vi "Add Item to Tree.vi"(6 "Display Text Override":string, 8 "error in (no error)":errorcluster, 9 "Parent Tag":string, 10 "Data Item":refnum<class "Data Item.lvclass">, 11 "Tree Manager in":refnum<class "Tree Manager.lvclass">) -> (0 "error out":errorcluster, 2 "New Tag":string, 3 "Tree Manager out":refnum<class "Tree Manager.lvclass">)   [LabVIEW 2026, in "VILab.lvlib" / "Tree Manager.lvclass"]
uses:
  Tree Manager.lvclass
  Data Item/Data Item.lvclass
  Tree Manager.lvclass/Tree Manager.ctl
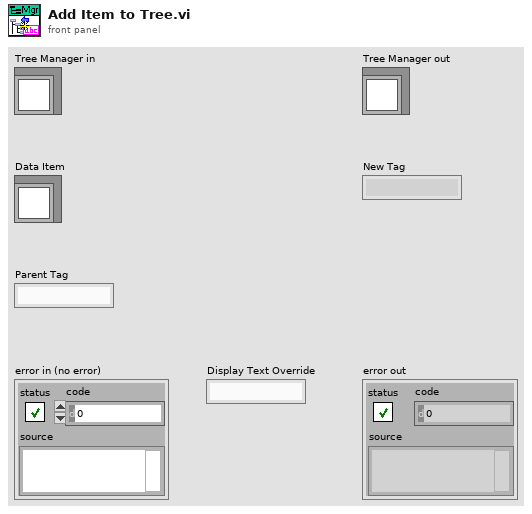
[diagram p1: front panel]
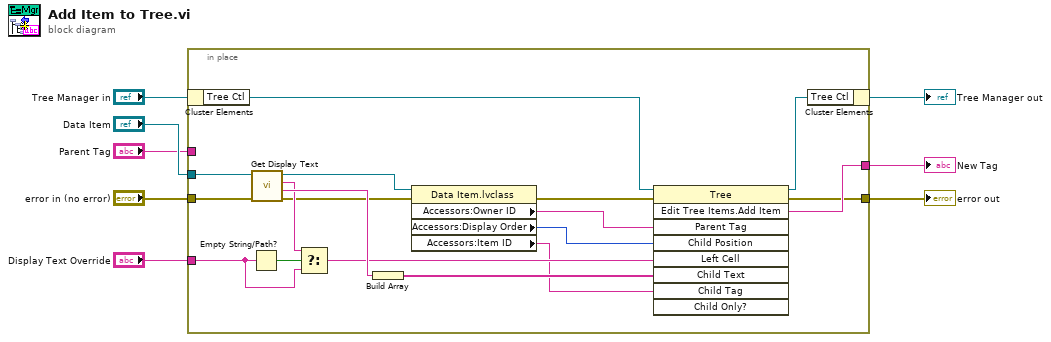
[diagram p0: block diagram]
diagram:
  n1 = in-place {
    in-place-border: "Data Item" -> [w25]
    in-place-border: "error in (no error)" -> [w26]
    in-place-border: "Parent Tag" -> [_]
    in-place-border: [w20] -> w2
    in-place-border: "Display Text Override" -> [w17]
    in-place-border: [w15] -> w7
    n2 = in-place-cluster #1("Tree Manager in") -> ("Tree Ctl"=w24:refnum<vi>)
    n3 = Empty String/Path?(string/path=w17) -> (empty?=w16:bool)
    n4 = call-dynamic "Get Display Text.vi"("error in (no error)"=w26, "Data Item in"=w25) -> ("error out"=w12:errorcluster, "Detail Text"=w23:string, "Display Name"=w18:string, "Data Item out"=w14:refnum<class "Data Item.lvclass">)  [unwired: 6 in]
    n5 = Select(t=w18, s=w16, f=w17) -> (s? t:f=w19:string)
    n6 = Build Array(w23) -> (w22:string[])
    n7 = property class="Data Item.lvclass"(reference=w14, error in=w12) -> (error out=w13:errorcluster, "Accessors:Owner ID"=w11:string, "Accessors:Display Order"=w10:i32, "Accessors:Item ID"=w9:string)  [unwired: 1 out]
    n8 = invoke class="Tree" method="Edit Tree Items.Add Item"(reference=w24, error in=w13, "Parent Tag"=w11, "Child Position"=w10, "Left Cell"=w19, "Child Text"=w22, "Child Tag"=w9) -> (reference out=w21:refnum<vi>, error out=w15:errorcluster, "Edit Tree Items:Add Item"=w20:string)  [unwired: 2 in, 6 out]
    n9 = in-place-cluster #1("Tree Ctl"=w21) -> (→"Tree Manager out":refnum<class "Tree Manager.lvclass">)
  }
  "error out" <- w7
  "New Tag" <- w2
